vi "esp301 set resetbeforemove.vi"(8 "error in (no error)":errorcluster, 9 "Args":string[](array[string]), 10 "String":string, 11 "ESP301 in":refnum<class "ESP301.lvclass">) -> (0 "error out":errorcluster, 2 "new commands":string, 3 "ESP301 out":refnum<class "ESP301.lvclass">)   [LabVIEW 2020, in "ESP301.lvclass"]
uses:
  ESP301.lvclass
  OnOffTypeDef.ctl
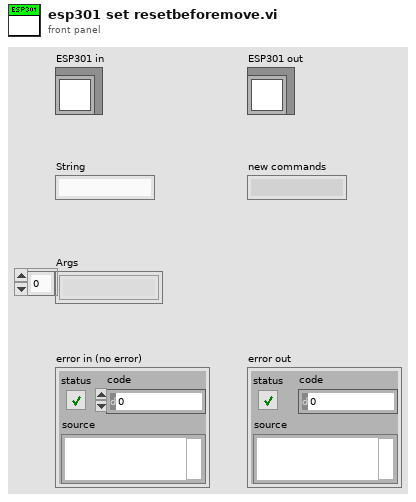
[diagram p1: front panel]
types:
  T1 = typedef "OnOffTypeDef.ctl" = enum16{"off", "on"}
  T2 = typedef "ESP301.lvclass/SettingsTypdef.ctl" = cluster{"devport":string, "Position":cluster{"Axis 1":cluster{"Value":dbl, "Min":dbl, "Max":dbl, "StepSize":dbl, "Tolerance":dbl, "ValueActual":dbl}, "Axis 2":cluster{"Value":dbl, "Min":dbl, "Max":dbl, "StepSize":dbl, "Tolerance":dbl, "ValueActual":dbl}, "Axis 3":cluster{"Value":dbl, "Min":dbl, "Max":dbl, "StepSize":dbl, "Tolerance":dbl, "ValueActual":dbl}}, "Power":cluster{"Axis 1":T1, "Axis 2":T1, "Axis 3":T1}, "Status":cluster{"Axis 1":T3, "Axis 2":T3, "Axis 3":T3}, "Backlash":cluster{"Axis 1":cluster{"Value":dbl, "Min":dbl, "Max":dbl, "StepSize":dbl, "Tolerance":dbl, "ValueActual":dbl}, "Axis 2":cluster{"Value":dbl, "Min":dbl, "Max":dbl, "StepSize":dbl, "Tolerance":dbl, "ValueActual":dbl}, "Axis 3":cluster{"Value":dbl, "Min":dbl, "Max":dbl, "StepSize":dbl, "Tolerance":dbl, "ValueActual":dbl}}, "Home":cluster{"Axis 1":cluster{"Value":dbl, "Min":dbl, "Max":dbl, "StepSize":dbl, "Tolerance":dbl, "ValueActual":dbl}, "Axis 2":cluster{"Value":dbl, "Min":dbl, "Max":dbl, "StepSize":dbl, "Tolerance":dbl, "ValueActual":dbl}, "Axis 3":cluster{"Value":dbl, "Min":dbl, "Max":dbl, "StepSize":dbl, "Tolerance":dbl, "ValueActual":dbl}}, "MoveToHardLimit":cluster{"Axis 1":T4, "Axis 2":T4, "Axis 3":T4}, "relativeMove":cluster{"Axis 1neg":T1, "Axis 2neg":T1, "Axis 3neg":T1, "Axis 1pos":T1, "Axis 2pos":T1, "Axis 3pos":T1}, "stepsize":cluster{"Value":dbl, "Min":dbl, "Max":dbl, "StepSize":dbl, "Tolerance":dbl, "ValueActual":dbl}, "automotoroff":T1, "ResetBeforeMove":T1, "Enable":cluster{"Axis 1":T1, "Axis 2":T1, "Axis 3":T1}}
  T3 = typedef "status_TypDef.ctl" = enum16{"Not referenced", "Homing", "Moving", "Ready"}
  T4 = typedef "Hardware limit.ctl" = enum16{"pos", "neg"}
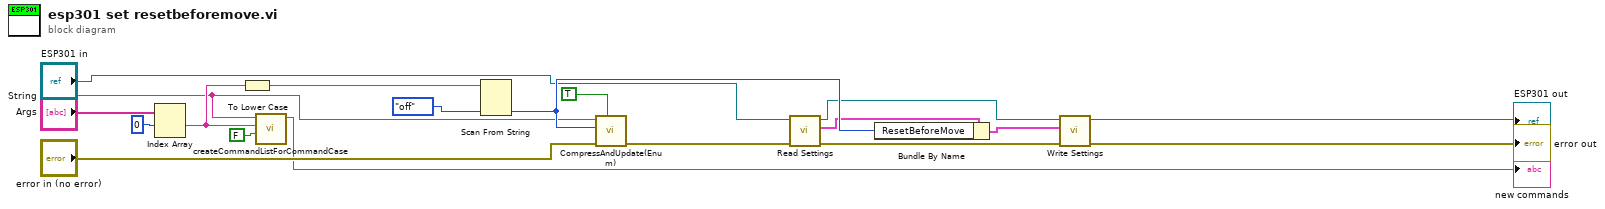
[diagram p0: block diagram]
diagram:
  n1 = Index Array(array="Args", index #1=0 ("number of group elements (0)")) -> (element #1=w8:string)  [unwired: 1 in, 1 out]
  n2 = To Lower Case(string=w8) -> (all lower case string=w4:string)
  n3 = call "createCommandListForCommandCase.vi"("immediate Check (only once)"=FALSE, "setvalue"=w8, "command"="String") -> ("new commands"=→"new commands":string)  [unwired: 8 in]
  n4 = Scan From String(input string=w4, default 1=OnOffTypeDef."off" ("Axis 1")) -> (output 1=w16:T1)  [unwired: 3 in, 3 out]
  n5 = call "CompressAndUpdate(Enum).vi"("force CVT update (false)"=TRUE ("force CVT update"), "error in"="error in (no error)", "enum variant"=w16, "command or variable name"="String") -> ("error out"=w18:errorcluster)  [unwired: 7 in]
  n6 = call-dynamic "Read Settings.vi"("error in (no error)"=w18, "ESP301 in"="ESP301 in") -> ("error out"=w13:errorcluster, "Settings"=w11:T2, "ESP301 out"=w10:refnum<class "ESP301.lvclass">)  [unwired: 7 in]
  n7 = Bundle By Name(cluster=w11, "ResetBeforeMove"=w16) -> (w12:T2)
  n8 = call-dynamic "Write Settings.vi"("error in (no error)"=w13, "Settings"=w12, "ESP301 in"=w10) -> ("error out"=→"error out":errorcluster, "ESP301 out"=→"ESP301 out":refnum<class "ESP301.lvclass">)  [unwired: 7 in]
